vi "Create Wheel by Type.vi"(8 "error in (no error)":errorcluster, 10 "wheel type":string) -> (0 "error out":errorcluster, 3 "wheel out":refnum<class "NI_Robotics_Wheel.lvclass">)   [LabVIEW 2017, in "NI_Robotics_Wheel.lvclass"]
uses:
  <vilib>/robotics/Steering/Wheel/NI_Robotics_Wheel.lvclass
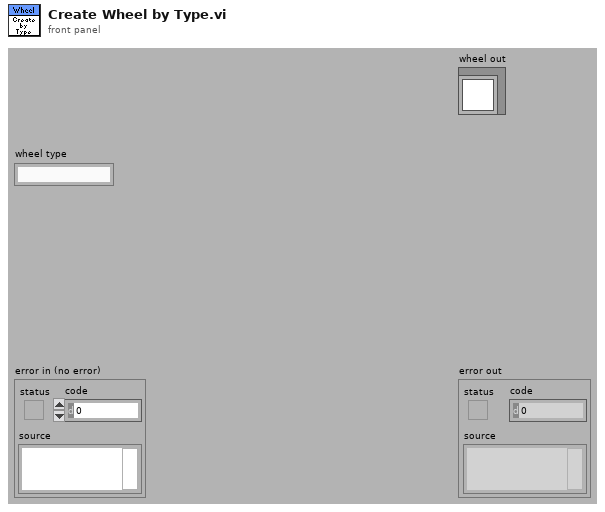
[diagram p1: front panel]
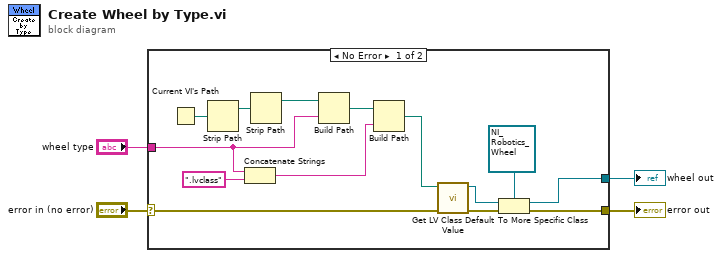
[diagram p0: block diagram]
diagram:
  n1 = case shown="No Error" "error in (no error)" {
    selector: "error in (no error)" -> [w10 w19]
    tunnel: [w6 w19] -> w3
    tunnel: "wheel type" -> [w14 _]
    tunnel: [w5 _] -> w1
    frame No Error {
      n2 = Current VI's Path() -> (path=w18:path)
      n3 = Strip Path(path=w18) -> (stripped path=w17:path)  [unwired: 1 out]
      n4 = Concatenate Strings(w14, ".lvclass" ("string")) -> (w12:string)
      n5 = Strip Path(path=w17) -> (stripped path=w15:path)  [unwired: 1 out]
      n6 = Build Path(base path=w15, name or relative path=w14) -> (appended path=w13:path)
      n7 = Build Path(base path=w13, name or relative path=w12) -> (appended path=w11:path)
      n8 = call <vilib>:"Get LV Class Default Value.vi"("error in (no error)"=w10, "class path"=w11) -> ("error out"=w9:errorcluster, "object"=w8:refnum<class>)  [unwired: 8 in]
      n9 = To More Specific Class(target class=refnum<class "NI_Robotics_Wheel.lvclass"> refnum ("RobotWheel out"), reference=w8, error in=w9) -> (specific class reference=w5:refnum<class "NI_Robotics_Wheel.lvclass">, error out=w6:errorcluster)
    }
    frame Error {
    }
  }
  "error out" <- w3
  "wheel out" <- w1
